vi "Drag Location.vi"(8 "error in (no error)":errorcluster, 9 "Coords":T4, 10 "BetterDropOp":refnum<class "BetterDropOp.lvclass">, 11 "BetterHandle in":refnum<class "BetterHandle.lvclass">) -> (0 "error out":errorcluster, 2 "DragOver Output":T1={"Displayed Row"=0, "Position"=enum."On Row", "Row's TreeItem index"=0, "indent"=0, "Accepted?"=FALSE, "Insertion index"=0, "Top left visible TreeItem index"=0, "Bar type"=enum."tilda up"}, 3 "BetterHandle out":refnum<class "BetterHandle.lvclass">)   [LabVIEW 2020, in "BetterDragAndDrop.lvlib" / "BetterHandle.lvclass"]
uses:
  BetterHandle.lvclass
  BetterDropOp/BetterDropOp.lvclass
  <vilib>/Utility/miscctls.llb/LVPoint32TypeDef.ctl
  SubVIs/DragOver Output.ctl
  SubVIs/DragOverPosition.ctl
  BetterTreeBar/SubVIs/Horizontal Bar Enumeration.ctl
  BetterTreeBar/BetterHorizontalBar.lvclass
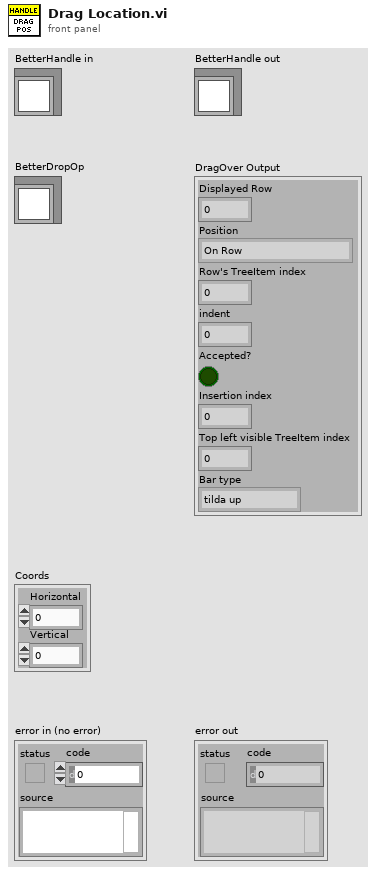
[diagram p1: front panel]
types:
  T1 = typedef "BetterDragAndDrop.lvlib/BetterHandle.lvclass/DragOver Output.ctl" = cluster{"Displayed Row":i32, "Position":T2, "Row's TreeItem index":i32, "indent":i32, "Accepted?":bool, "Insertion index":i32, "Top left visible TreeItem index":i32, "Bar type":T3}
  T2 = typedef "BetterDragAndDrop.lvlib/BetterHandle.lvclass/DragOverPosition.ctl" = enum16{"On Row", "Inbetween"}
  T3 = typedef "BetterDragAndDrop.lvlib/BetterHorizontalBar.lvclass/Horizontal Bar Enumeration.ctl" = enum16{"None", "only bar", "tilda up"}
  T4 = typedef "LVPoint32TypeDef.ctl" = cluster{"Horizontal":i32, "Vertical":i32}
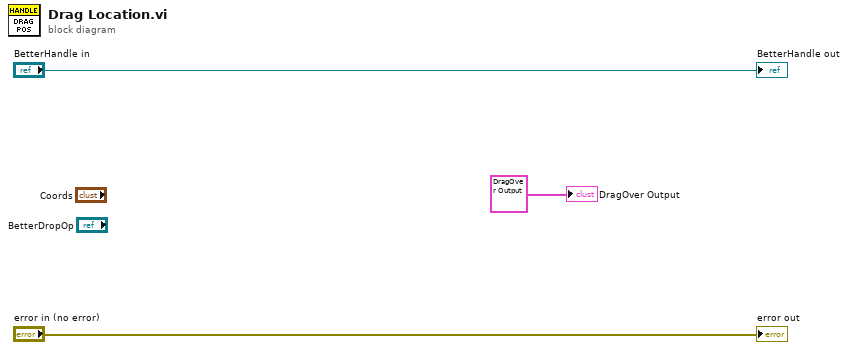
[diagram p0: block diagram]
diagram:
  "error out" <- "error in (no error)"
  "BetterHandle out" <- "BetterHandle in"
  "DragOver Output" <- T1 {"Displayed Row"=0, "Position"=enum."On Row", "Row's TreeItem index"=0, "indent"=0, "Accepted?"=FALSE, "Insertion index"=0, "Top left visible TreeItem index"=0, "Bar type"=enum."tilda up"} ("DragOver Output")
